vi "ClimbBegin.vi"(8 "error in (no error)":errorcluster) -> (0 "error out":errorcluster)   [LabVIEW 2023]
uses:
  <vilib>/Rock Robotics/WPI/ThirdParty/REV Robotics/REVLib/Typedef/Spark MAX Sensor Type.ctl
  <vilib>/Rock Robotics/WPI/ThirdParty/REV Robotics/REVLib/Typedef/Spark MAX Limit Switch Polarity.ctl
  <vilib>/Rock Robotics/WPI/ThirdParty/REV Robotics/REVLib/Typedef/Spark MAX Limit Direction.ctl
  <vilib>/Rock Robotics/WPI/ThirdParty/REV Robotics/REVLib/Typedef/Spark MAX Idle Mode.ctl
  <vilib>/Rock Robotics/WPI/ThirdParty/REV Robotics/REVLib/Typedef/Spark MAX Motor Type.ctl
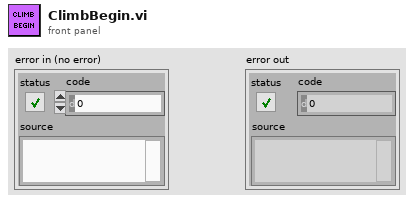
[diagram p1: front panel]
types:
  T1 = typedef "Spark MAX Sensor Type.ctl" = enum16{"No Sensor", "Hall Sensor", "Encoder", "-Not Available-", "Analog", "Alternate Encoder", "Duty Cycle"}
  T2 = typedef "Spark MAX Limit Switch Polarity.ctl" = enum16{"Normally Open", "Normally Closed"}
  T3 = typedef "Spark MAX Limit Direction.ctl" = enum16{"Forward Limit", "Reverse Limit"}
  T4 = typedef "Spark MAX Idle Mode.ctl" = enum16{"Coast", "Brake"}
  T5 = typedef "Spark MAX Motor Type.ctl" = enum16{"Brushed", "Brushless"}
  T6 = typedef "WPI_MotorControlDeviceRef.ctl" = cluster{"DeviceStatus":errorcluster, "Type":T7, "PWM":cluster{"PWM Channel":T8, "DeadBand":T9}, "CAN":cluster{"Device Number":u8, "SetOutput VI Ref":variant, "GetOutput VI Ref":variant, "Enable VI Ref":variant, "Disable VI Ref":variant, "Data":variant}, "Invert":bool, "DIO PWM":cluster{"PWM \"Enable\" Channel":T8, "DIOChannel":T10, "PWM Rate":dbl}}
  T7 = typedef "WPI_MotorControlType.ctl" = enum16{"PWM", "CAN", "DIO PWM"}
  T8 = typedef "FPGA_DIOPWMChannel.ctl" = enum8{"PWM 0", "PWM 1", "PWM 2", "PWM 3", "PWM 4", "PWM 5", "PWM 6", "PWM 7", "PWM 8", "PWM 9", "PWM MXP 0", "PWM MXP 1", "PWM MXP 2", "PWM MXP 3", "PWM MXP 4", "PWM MXP 5", "PWM MXP 6", "PWM MXP 7", "PWM MXP 8", "PWM MXP 9", "Invalid"}
  T9 = typedef "WPI_PWMDeadband.ctl" = cluster{"Name":string, "maxPositivePwm":i32, "minPositivePwm":i32, "centerPwm":i32, "maxNegativePwm":i32, "minNegativePwm":i32, "angularRange":u16}
  T10 = typedef "FPGA_DIOChannel.ctl" = enum8{"DIO 0", "DIO 1", "DIO 2", "DIO 3", "DIO 4", "DIO 5", "DIO 6", "DIO 7", "DIO 8", "DIO 9", "DIO MXP 0", "DIO MXP 1", "DIO MXP 2", "DIO MXP 3", "DIO MXP 4", "DIO MXP 5", "DIO MXP 6", "DIO MXP 7", "DIO MXP 8", "DIO MXP 9", "DIO MXP 10", "DIO MXP 11", "DIO MXP 12", "DIO MXP 13", "DIO MXP 14", "DIO MXP 15", "SPI Port CS1", "SPI Port CS2", "SPI Port CS3", "SPI Port MISO", "SPI Port MOSI", "Invalid"}
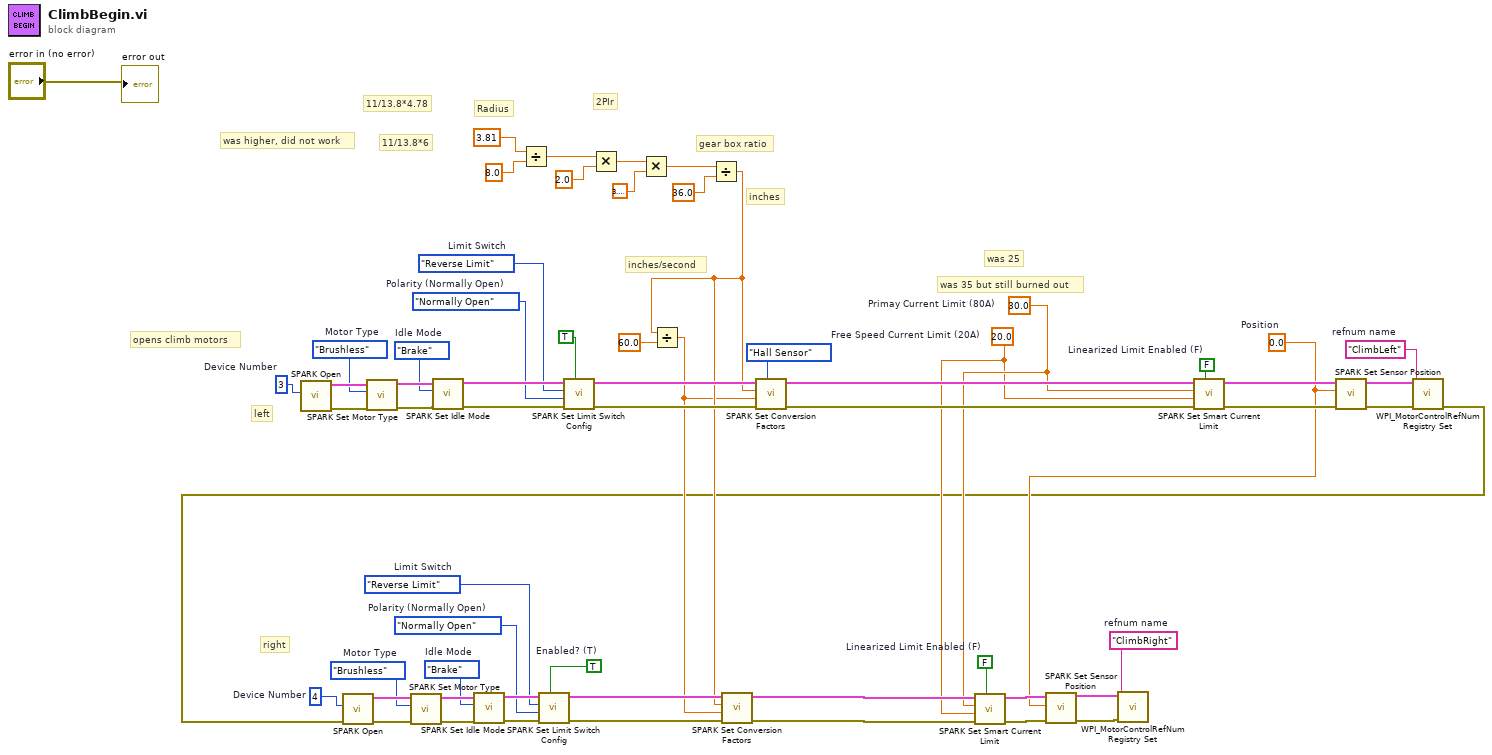
[diagram p0: block diagram]
diagram:
  w1 = FALSE  # Linearized Limit Enabled (F)
  w2 = FALSE  # Linearized Limit Enabled (F)
  w10 = 0.0  # Position
  w28 = TRUE  # Enabled? (T)
  w5 = 20.0  # Free Speed Current Limit (20A)
  w6 = 30.0  # Primay Current Limit (80A)
  w30 = Spark_MAX_Limit_Switch_Polarity."Normally Open"  # Polarity (Normally Open)
  w31 = Spark_MAX_Limit_Direction."Reverse Limit"  # Limit Switch
  w32 = Spark_MAX_Limit_Switch_Polarity."Normally Open"  # Polarity (Normally Open)
  w33 = Spark_MAX_Limit_Direction."Reverse Limit"  # Limit Switch
  w43 = Spark_MAX_Idle_Mode."Brake"  # Idle Mode
  w44 = Spark_MAX_Idle_Mode."Brake"  # Idle Mode
  w47 = Spark_MAX_Motor_Type."Brushless"  # Motor Type
  w48 = Spark_MAX_Motor_Type."Brushless"  # Motor Type
  w49 = "ClimbRight"  # refnum name
  w50 = "ClimbLeft"  # refnum name
  w54 = u8 4  # Device Number
  w55 = u8 3  # Device Number
  # "was 35 but still burned out"
  # "11/13.8*4.78"
  # "was higher, did not work"
  # "11/13.8*6"
  # "was 25"
  # "inches/second"
  # "inches"
  # "gear box ratio"
  # "2PIr"
  # "Radius"
  # "opens climb motors"
  # "right"
  # "left"
  n1 = call <vilib>:"SPARK Open.vi"("Device Number"=w55) -> ("error out"=w56:errorcluster, "MotorControlDeviceRef"=w57:T6)  [unwired: 9 in]
  n2 = call <vilib>:"SPARK Set Motor Type.vi"("error in (no error)"=w56, "Motor Type"=w48, "MotorControlDevRef"=w57) -> ("error out"=w42:errorcluster, "MotorControlDeviceRef"=w46:T6)  [unwired: 7 in]
  n3 = call <vilib>:"SPARK Set Idle Mode.vi"("error in (no error)"=w42, "Idle Mode"=w43, "MotorControlDeviceRef in"=w46) -> ("error out"=w34:errorcluster, "MotorControlDeviceRef out"=w35:T6)  [unwired: 7 in]
  n4 = Divide(x=3.81, y=8.0) -> (x/y=w20:dbl)
  n5 = call <vilib>:"SPARK Set Limit Switch Config.vi"("Enabled? (T)"=TRUE, "error in (no error)"=w34, "Polarity (Normally Open)"=w32, "Limit Switch"=w33, "MotorControlDeviceRef in"=w35) -> ("error out"=w25:errorcluster, "MotorControlDeviceRef out"=w27:T6)  [unwired: 5 in]
  n6 = Multiply(x=w20, y=2.0) -> (x*y=w18:dbl)
  n7 = Multiply(x=w18, y=3.141592653589793) -> (x*y=w16:dbl)
  n8 = Divide(x=w16, y=36.0) -> (x/y=w8:dbl)
  n9 = Divide(x=w8, y=60.0) -> (x/y=w7:dbl)
  n10 = call <vilib>:"SPARK Set Conversion Factors.vi"("Sensor Type (Hall Sensor)"=Spark_MAX_Sensor_Type."Hall Sensor", "error in (no error)"=w25, "Velocity Factor (1)"=w7, "Position Factor (1)"=w8, "MotorControlDeviceRef in"=w27) -> ("error out"=w24:errorcluster, "MotorControlDeviceRef out"=w26:T6)  [unwired: 5 in]
  n11 = call <vilib>:"SPARK Set Smart Current Limit.vi"("Linearized Limit Enabled (F)"=w2, "error in (no error)"=w24, "Free Speed Current Limit (20A)"=w5, "Primay Current Limit (80A)"=w6, "MotorControlDeviceRef in"=w26) -> ("error out"=w61:errorcluster, "MotorControlDeviceRef out"=w60:T6)  [unwired: 5 in]
  n12 = call <vilib>:"SPARK Set Sensor Position.vi"("error in"=w61, "Position"=w10, "MotorControlDeviceRef"=w60) -> ("error out"=w41:errorcluster, "MotorControlDeviceRef"=w52:T6)  [unwired: 7 in]
  n13 = call <vilib>:"WPI_MotorControlRefNum Registry Set.vi"("error in (no error)"=w41, "refnum name"=w50, "MotorControlDevRef"=w52) -> ("error out"=w3:errorcluster)  [unwired: 7 in, 1 out]
  n14 = call <vilib>:"SPARK Open.vi"("error in (no error)"=w3, "Device Number"=w54) -> ("error out"=w40:errorcluster, "MotorControlDeviceRef"=w53:T6)  [unwired: 8 in]
  n15 = call <vilib>:"SPARK Set Motor Type.vi"("error in (no error)"=w40, "Motor Type"=w47, "MotorControlDevRef"=w53) -> ("error out"=w39:errorcluster, "MotorControlDeviceRef"=w45:T6)  [unwired: 7 in]
  n16 = call <vilib>:"SPARK Set Idle Mode.vi"("error in (no error)"=w39, "Idle Mode"=w44, "MotorControlDeviceRef in"=w45) -> ("error out"=w36:errorcluster, "MotorControlDeviceRef out"=w37:T6)  [unwired: 7 in]
  n17 = call <vilib>:"SPARK Set Limit Switch Config.vi"("Enabled? (T)"=w28, "error in (no error)"=w36, "Polarity (Normally Open)"=w30, "Limit Switch"=w31, "MotorControlDeviceRef in"=w37) -> ("error out"=w12:errorcluster, "MotorControlDeviceRef out"=w14:T6)  [unwired: 5 in]
  n18 = call <vilib>:"SPARK Set Conversion Factors.vi"("error in (no error)"=w12, "Velocity Factor (1)"=w7, "Position Factor (1)"=w8, "MotorControlDeviceRef in"=w14) -> ("error out"=w11:errorcluster, "MotorControlDeviceRef out"=w13:T6)  [unwired: 6 in]
  n19 = call <vilib>:"SPARK Set Smart Current Limit.vi"("Linearized Limit Enabled (F)"=w1, "error in (no error)"=w11, "Free Speed Current Limit (20A)"=w5, "Primay Current Limit (80A)"=w6, "MotorControlDeviceRef in"=w13) -> ("error out"=w59:errorcluster, "MotorControlDeviceRef out"=w58:T6)  [unwired: 5 in]
  n20 = call <vilib>:"SPARK Set Sensor Position.vi"("error in"=w59, "Position"=w10, "MotorControlDeviceRef"=w58) -> ("error out"=w38:errorcluster, "MotorControlDeviceRef"=w51:T6)  [unwired: 7 in]
  n21 = call <vilib>:"WPI_MotorControlRefNum Registry Set.vi"("error in (no error)"=w38, "refnum name"=w49, "MotorControlDevRef"=w51) -> ()  [unwired: 7 in, 2 out]
  "error out" <- "error in (no error)"
